vi "Add Items.vi"(7 "Mode":enum16{"End", "Begin"}(ring), 8 "错误输入":errorcluster, 10 "Items":string[](array[string]), 11 "Listbox Ref":refnum<vi>) -> (0 "错误输出":errorcluster, 3 "Dup Listbox Ref":refnum<vi>)   [LabVIEW 2012, in "Listbox Tool.lvlib"]
uses:
  Listbox Tool.lvlib
  Custom Type/Read and Write Mode.ctl
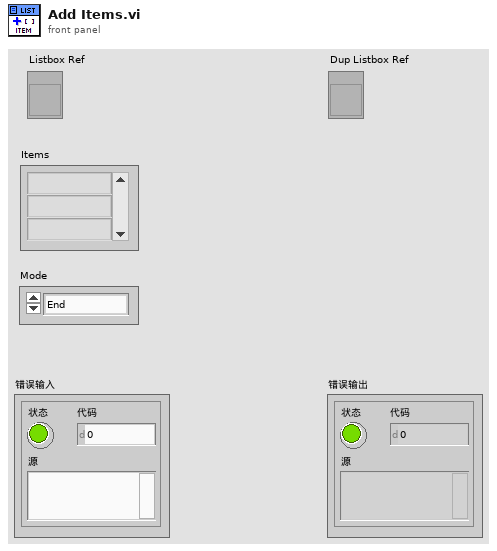
[diagram p1: front panel]
types:
  T1 = typedef "Listbox Tool.lvlib/Read and Write Mode.ctl" = enum16{"Read", "Write"}
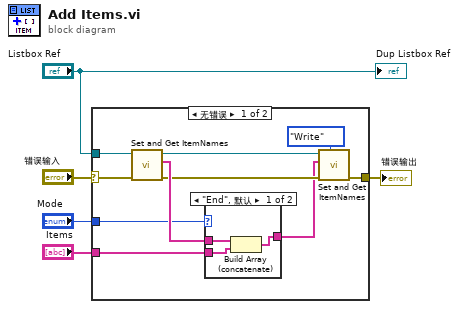
[diagram p0: block diagram]
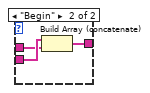
[diagram p2: hidden frame]
diagram:
  n1 = case shown="无错误" "错误输入" {
    selector: "错误输入" -> [w15 w22]
    tunnel: "Listbox Ref" -> [w14 _]
    tunnel: "Items" -> [w12 _]
    tunnel: "Mode" -> [w7 _]
    tunnel: [w6 w22] -> w1
    frame No Error {
      n2 = call "Set and Get ItemNames.vi"("错误输入"=w15, "Listbox Ref"=w14) -> ("错误输出"=w11:errorcluster, "ItemNames Out"=w13:string[], "Dup Listbox Ref"=w9:refnum<vi>)  [unwired: 7 in]
      n3 = case shown="\"End\", 默认" w7 {
        tunnel: w13 -> [w18 w20]
        tunnel: w12 -> [w17 w21]
        tunnel: [w16 w19] -> w10
        frame "End", Default {
          n4 = Build Array (concatenate)(w18, w17) -> (w16:string[])
        }
        frame "Begin" {
          n5 = Build Array (concatenate)(w21, w20) -> (w19:string[])
        }
      }
      n6 = call "Set and Get ItemNames.vi"("Mode"=Read_and_Write_Mode."Write", "错误输入"=w11, "ItemNames In"=w10, "Listbox Ref"=w9) -> ("错误输出"=w6:errorcluster)  [unwired: 5 in, 2 out]
    }
    frame Error {
    }
  }
  "错误输出" <- w1
  "Dup Listbox Ref" <- "Listbox Ref"
